vi "401_LV2G_DB.vi"(8 "error in (no error)":errorcluster, 11 "Action":enum16{"Open", "Read", "Close"}(ring)) -> (0 "error out":errorcluster, 3 "DB_Ref":T1)   [LabVIEW 2015]
uses:
  <vilib>/addons/database/Connection.llb/Conn ObjectReference.ctl
  <vilib>/addons/database/Connection.llb/DB Tools Open Connec (String).vi
  <vilib>/addons/database/NI_Database_API.lvlib
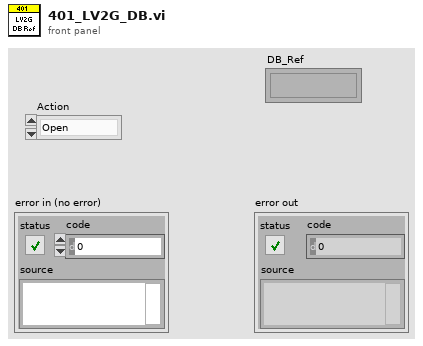
[diagram p1: front panel]
types:
  T1 = typedef "NI_Database_API.lvlib/Conn ObjectReference.ctl" = refnum<k1>
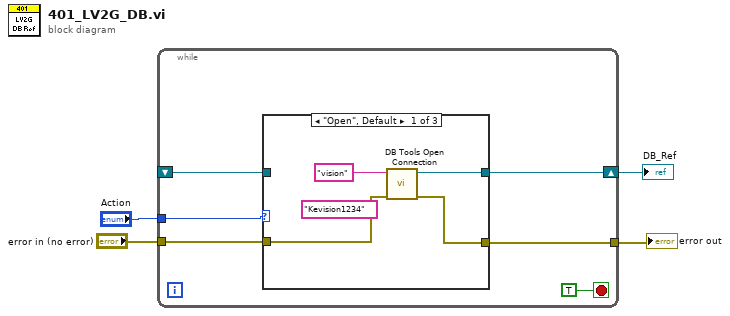
[diagram p0: block diagram]
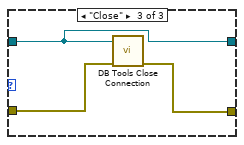
[diagram p3: hidden frame]
diagram:
  n1 = while {
    tunnel: "Action" -> [w9]
    shift-right: [w8] -> w1
    shift-left: _ -> [w7]
    tunnel: "error in (no error)" -> [w6]
    tunnel: [w5] -> w2
    stop <- TRUE stop-if-true
    n2 = case shown="\"Open\", Default" w9 {
      tunnel: [w13 w16 w19] -> w8
      tunnel: w7 -> [_ w16 w19]
      tunnel: w6 -> [w12 w15 w17]
      tunnel: [w11 w15 w18] -> w5
      frame "Open", Default {
        (unwired) "Kevision1234" ("password")
        n3 = call-poly <vilib>:"DB Tools Open Connection.vi"("error in (no error)"=w12, "connection information"="vision" ("userID")) -> ("error out"=w11:errorcluster, "connection reference"=w13:T1)  [unwired: 6 in]
      }
      frame "Read" {
      }
      frame "Close" {
        n4 = call <vilib>:"DB Tools Close Connection.vi"("error in (no error)"=w17, "connection reference"=w19) -> ("error out"=w18:errorcluster)  [unwired: 5 in]
      }
    }
  }
  "error out" <- w2
  "DB_Ref" <- w1
